vi "debug_clear_myrioFolder.vi"() -> ()   [LabVIEW 2014]
panel:
  out "error out":errorcluster
  out "error in 3":errorcluster
  out "error in 2":errorcluster
  in  "error in":errorcluster
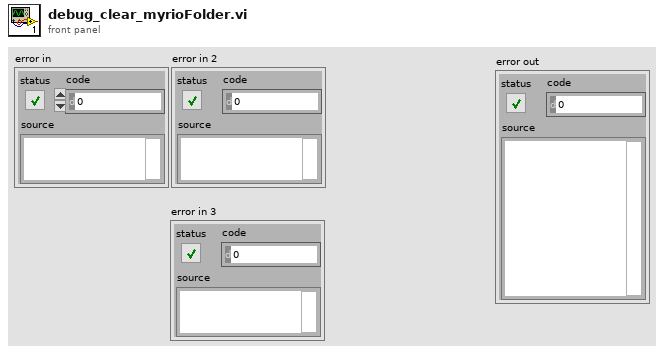
[diagram p1: front panel]
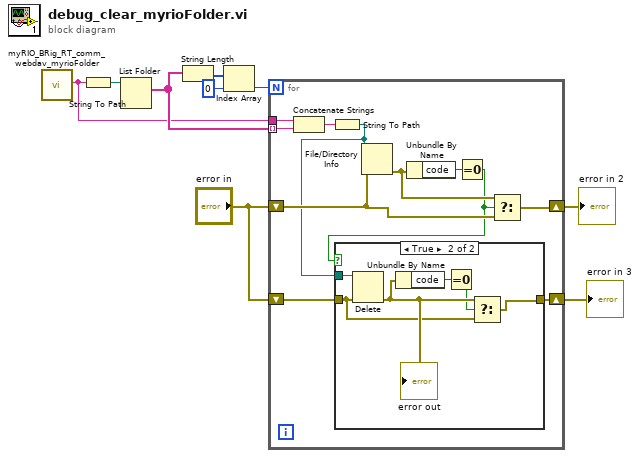
[diagram p0: block diagram]
diagram:
  n1 = call "myRIO_BRig_RT_comm_webdav_myrioFolder.vi"() -> ("output_myrioFolder"=w5:string)  [unwired: 11 in]
  n2 = String To Path(string=w5) -> (path=w2:path)
  n3 = List Folder(path=w2) -> (filenames=w6:string[])  [unwired: 3 in, 3 out]
  n4 = String Length(string=w6) -> (length=w9:i32[])
  n5 = Index Array(array=w9, index=0) -> (element=w7:i32)
  n6 = for {
    N: w7 -> [_]
    tunnel: w6 -> [w20] mode=indexing
    tunnel: w5 -> [w19]
    shift-right: [w14] -> w4
    shift-left: "error in" -> [w15]
    shift-right: [w12] -> w1
    shift-left: "error in" -> [w10]
    n7 = Concatenate Strings(w19, w20) -> (w18:string)
    n8 = String To Path(string=w18) -> (path=w11:path)
    n9 = File/Directory Info(path=w11, error in=w15) -> (error out=w16:errorcluster)  [unwired: 6 out]
    n10 = Unbundle By Name(w16) -> ("code"=w17:i32)
    n11 = Equal To 0?(x=w17) -> (x = 0?=w13:bool)
    n12 = case shown="True" w13 {
      tunnel: w11 -> [_ w27]
      tunnel: [w21 w24] -> w12
      tunnel: w10 -> [w21 w22]
      frame False {
      }
      frame True {
        n13 = Delete(path (use dialog)=w27, error in=w22) -> (error out=w25:errorcluster)  [unwired: 3 in, 2 out]
        "error out" <- w25
        n14 = Unbundle By Name(w25) -> ("code"=w26:i32)
        n15 = Equal To 0?(x=w26) -> (x = 0?=w23:bool)
        n16 = Select(t=w25, s=w23, f=w22) -> (s? t:f=w24:errorcluster)
      }
    }
    n17 = Select(t=w16, s=w13, f=w15) -> (s? t:f=w14:errorcluster)
  }
  "error in 2" <- w4
  "error in 3" <- w1
